vi "Configure RF Squelch.vi"(7 "Enable Squelch (T: Enable)":bool=TRUE, 8 "error in (no error)":errorcluster, 10 "Squelch Threshold (1V)":dbl=1.0 min=0.0 max=40.0 step=0.1 format="%#_g V", 11 "VISA resource name":refnum<visa-resource-name>) -> (0 "error out":errorcluster, 3 "VISA resource name out":refnum<visa-resource-name>)   [LabVIEW 2017, in "Scope.lvlib" / "Tektronix DPO MSO 2000 4000 Series.lvlib"]
doc: "Configures the parameters for the Squelch function of MDO series oscillocopes.\n\n<B>Note:</B>\n- The Frequency or Phase RF channels must be enabled to use this VI. The Frequency Channel will become enabled if both channels are disabled when this VI is run.\n-This VI is only applicable to <B>MDO4000 series</B> oscilloscopes."
uses:
  Tektronix DPO MSO 2000 4000 Series.lvlib
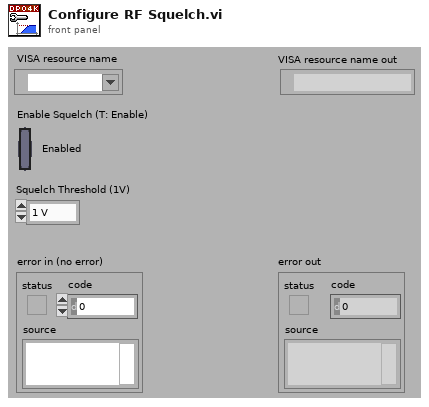
[diagram p1: front panel]
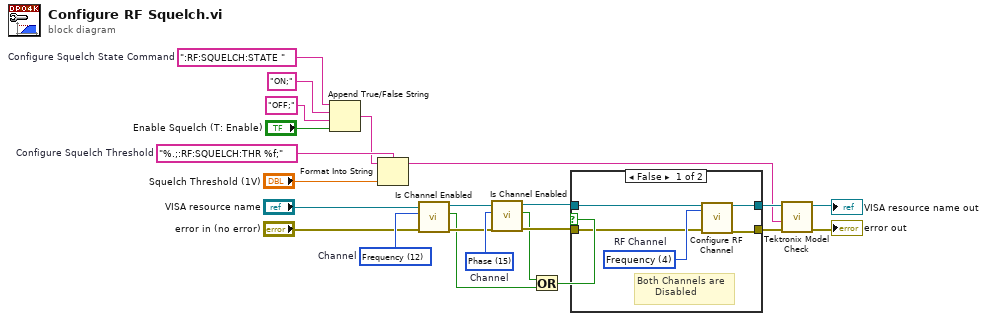
[diagram p0: block diagram]
diagram:
  w11 = u16 15 items=["Channel 1", "Channel 2", "Channel 3", "Channel 4", "Math", "Reference 1", "Reference 2", "Reference 3", "Reference 4", "Normal", "Average", "Amplitude", "Frequency", "Minimum Peak Hold", "Maximum Peak Hold", "Phase"]  # Channel
  w14 = u16 12 items=["Channel 1", "Channel 2", "Channel 3", "Channel 4", "Math", "Reference 1", "Reference 2", "Reference 3", "Reference 4", "Normal", "Average", "Amplitude", "Frequency", "Minimum Peak Hold", "Maximum Peak Hold", "Phase"]  # Channel
  w18 = "%.;:RF:SQUELCH:THR %f;"  # Configure Squelch Threshold
  w22 = ":RF:SQUELCH:STATE "  # Configure Squelch State Command
  n1 = Append True/False String(1:"Enable Squelch (T: Enable)", 2:"OFF;" ("false string"), 3:"ON;" ("true string"), 4:w22) -> (0:w17:string)
  n2 = Format Into String(format string=w18, initial string=w17, "Squelch Threshold (1V)") -> (resulting string=w7:string)  [unwired: 1 in, 1 out]
  n3 = call "Is Channel Enabled.vi"("error in (no error)"="error in (no error)", "Channel (0: Channel 1)"=w14, "VISA resource name"="VISA resource name") -> ("error out"=w5:errorcluster, "Enabled"=w2:bool, "VISA resource name out"=w6:refnum<visa-resource-name>)  [unwired: 6 in]
  n4 = call "Is Channel Enabled.vi"("error in (no error)"=w5, "Channel (0: Channel 1)"=w11, "VISA resource name"=w6) -> ("error out"=w3:errorcluster, "Enabled"=w1:bool, "VISA resource name out"=w4:refnum<visa-resource-name>)  [unwired: 6 in]
  n5 = Or(x=w1, y=w2) -> (x .or. y?=w10:bool)
  n6 = case shown="False" w10 {
    tunnel: w3 -> [w26 w29]
    tunnel: w4 -> [w27 w30]
    tunnel: [w25 w30] -> w9
    tunnel: [w24 w29] -> w8
    frame False {
      w28 = u16 4 items=["Normal", "Average", "Amplitude", "Phase", "Frequency", "Maximum Peak Hold", "Minimum Peak Hold"]  # RF Channel
      # "Both Channels are\n      Disabled"
      n7 = call "Configure RF Channel.vi"("VISA resource name"=w27, "RF Channel (0:Normal)"=w28, "error in (no error)"=w26) -> ("VISA resource name out"=w25:refnum<visa-resource-name>, "error out"=w24:errorcluster)  [unwired: 15 in]
    }
    frame True {
      # "Either the Frequency\nor Phase channel\n     is enabled"
    }
  }
  n8 = call "Tektronix Model Check.vi"("error in (no error)"=w8, "Command String"=w7, "VISA resource name"=w9) -> ("error out"=→"error out":errorcluster, "VISA resource name out"=→"VISA resource name out":refnum<visa-resource-name>)  [unwired: 7 in]
